vi "Identify Cryo-Con.vi"(8 "Error In":errorcluster, 11 "VISA resource name":refnum<visa-resource-name>) -> (0 "Error Out":errorcluster, 1 "data string out":string, 2 "Cryo-con":bool, 3 "VISA resource name out":refnum<visa-resource-name>)   [LabVIEW 2016]
uses:
  GPIB/VISA  Send Receive.vi
panel:
  in  "Serial Configuration":cluster{"Baud Rate":u32}={"Baud Rate"=9600} {"Baud Rate" items=["300"=300, "600"=600, "1200"=1200, "2400"=2400, "4800"=4800, "9600"=9600, "19200"=19200]}
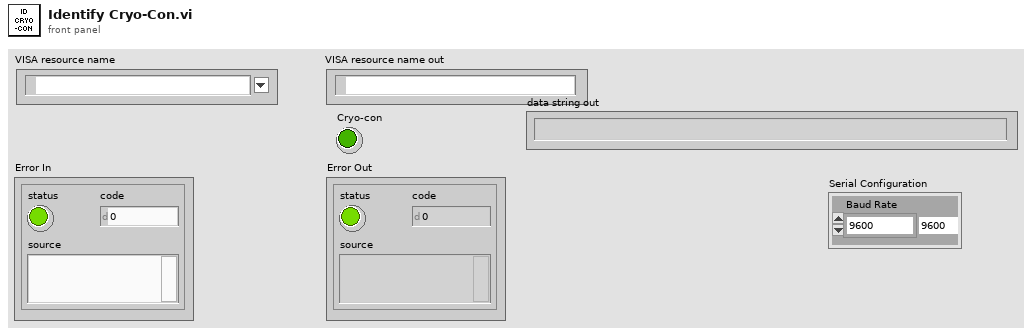
[diagram p1: front panel]
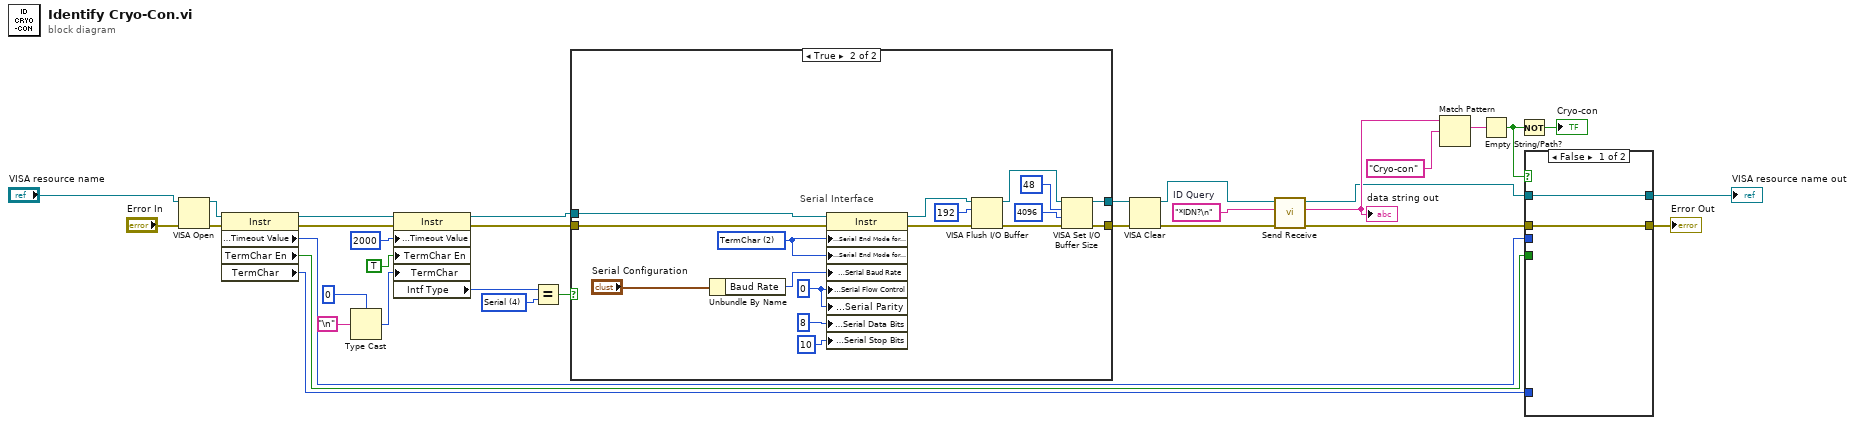
[diagram p0: block diagram]
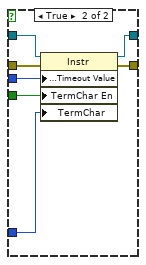
[diagram p3: hidden frame]
diagram:
  w7 = u16 4 items=["GPIB"=1, "VXI"=2, "GPIB-VXI"=3, "Serial"=4, "PXI"=5, "TCPIP"=6, "USB"=7] ("Interface Information:Interface Type")
  w22 = "*IDN?\n"  # ID Query
  n1 = VISA Open(error in (no error)="Error In", VISA resource name="VISA resource name") -> (VISA resource name=w24:refnum<visa-resource-name>, error out=w25:errorcluster)  [unwired: 3 in]
  n2 = property class="Instr"(reference=w24, error in=w25) -> (reference out=w23:refnum<visa-resource-name>, error out=w26:errorcluster, "General Settings:Timeout Value"=w14:u32, "TermChar En"=w13:bool, "TermChar"=w12:u8)
  n3 = Type Cast(type=u8 0, x="\n" ("Line Feed Constant")) -> (*(type *) &x=w33:u8)
  n4 = property class="Instr"(reference=w23, error in=w26, "General Settings:Timeout Value"=u32 2000, "TermChar En"=TRUE ("Message Based Settings:Termination Character Enable"), "TermChar"=w33) -> (reference out=w3:refnum<visa-resource-name>, error out=w5:errorcluster, "Intf Type"=w4:u16)
  n5 = Equal?(x=w4, y=w7) -> (x = y?=w6:bool)
  n6 = case shown="True" w6 {
    tunnel: [w34 w49] -> w2
    tunnel: [w35 w46] -> w1
    tunnel: w3 -> [w34 w51]
    tunnel: w5 -> [w35 w52]
    frame False {
      # "TCP/IP uses end-of-line char of \\n to terminate reads"
      # "GPIB and TCP/IP Interfaces"
    }
    frame True {
      w38 = u16 0
      w41 = u16 2 items=["None", "LastBit", "TermChar"] ("Serial Settings:Serial End Mode for Reads")
      # "Serial Interface"
      n7 = Unbundle By Name("Serial Configuration") -> ("Baud Rate"=w40:u32)
      n8 = property class="Instr"(reference=w51, error in=w52, "Serial Settings:Serial End Mode for Reads"=w41, "Serial Settings:Serial End Mode for Writes"=w41, "Serial Settings:Serial Baud Rate"=w40, "Serial Settings:Serial Flow Control"=w38, "Serial Settings:Serial Parity"=w38, "Serial Settings:Serial Data Bits"=u16 8, "Serial Settings:Serial Stop Bits"=u16 10) -> (reference out=w45:refnum<visa-resource-name>, error out=w48:errorcluster)
      n9 = VISA Flush I/O Buffer(VISA resource name=w45, mask (16)=u16 192, error in (no error)=w48) -> (VISA resource name out=w50:refnum<visa-resource-name>, error out=w47:errorcluster)
      n10 = VISA Set I/O Buffer Size(VISA resource name=w50, mask (16)=u16 48, size (4096)=u32 4096 ("size (0)"), error in (no error)=w47) -> (VISA resource name out=w49:refnum<visa-resource-name>, error out=w46:errorcluster)
    }
  }
  n11 = VISA Clear(VISA resource name=w2, error in (no error)=w1) -> (VISA resource name out=w9:refnum<visa-resource-name>, error out=w8:errorcluster)
  n12 = call-poly "Send Receive.vi"("error in (no error)"=w8, "data string in"=w22, "VISA Resource Name"=w9) -> ("error out"=w16:errorcluster, "data string out"=w21:string, "VISA Resource Name Out"=w15:refnum<visa-resource-name>)  [unwired: 6 in]
  "data string out" <- w21
  n13 = Match Pattern(string=w21, regular expression="Cryo-con") -> (match substring=w19:string)  [unwired: 1 in, 3 out]
  n14 = Empty String/Path?(string/path=w19) -> (empty?=w17:bool)
  n15 = Not(x=w17) -> (.not. x?=→"Cryo-con":bool)
  n16 = case shown="False" w17 {
    tunnel: w16 -> [w54 w60]
    tunnel: w15 -> [w53 w61]
    tunnel: w14 -> [_ w59]
    tunnel: w13 -> [_ w58]
    tunnel: w12 -> [_ w57]
    tunnel: [w54 w56] -> w11
    tunnel: [w53 w55] -> w10
    frame False {
    }
    frame True {
      n17 = property class="Instr"(reference=w61, error in=w60, "General Settings:Timeout Value"=w59, "TermChar En"=w58, "TermChar"=w57) -> (reference out=w55:refnum<visa-resource-name>, error out=w56:errorcluster)
    }
  }
  "VISA resource name out" <- w10
  "Error Out" <- w11
